vi "getEngineeringStatus.vi"(8 "error in (no error)":errorcluster, 11 "DomeCommunicator in":refnum<class "DomeCommunicator.lvclass">) -> (0 "error out":errorcluster, 1 "timeout":bool, 2 "fullEngineeringStatus":T1 {"shortStatus"."azimuthAngle" min=0.0 max=360.0; "shortStatus"."dropoutDoorOpeningPercentage" min=0.0 max=100.0; "shortStatus"."mainDoorOpeningPercentage" min=0.0 max=100.0}, 3 "DomeCommunicator out":refnum<class "DomeCommunicator.lvclass">, 4 "response":string)   [LabVIEW 2016, in "DomeCommunicator.lvclass"]
uses:
  DomeCommunicator.lvclass
  ComTypedefs/fullEngineeringStatus.ctl
  ComTypedefs/shortStatus.ctl
  ComTypedefs/openingStates.ctl
  IDome/domeTypedefs/openingPercentage.ctl
  ComTypedefs/sensorCode.ctl
  ComTypedefs/azimimuthPositionStatus.ctl
  IDome/domeTypedefs/azimuth.ctl
  IDome/domeTypedefs/direction.ctl
  IDome/domeTypedefs/domeState.ctl
  IDome/domeTypedefs/motionDirection.ctl
  IDome/domeTypedefs/openingMotion.ctl
  ComTypedefs/engineeringStatus.ctl
  ComTypedefs/queries.ctl
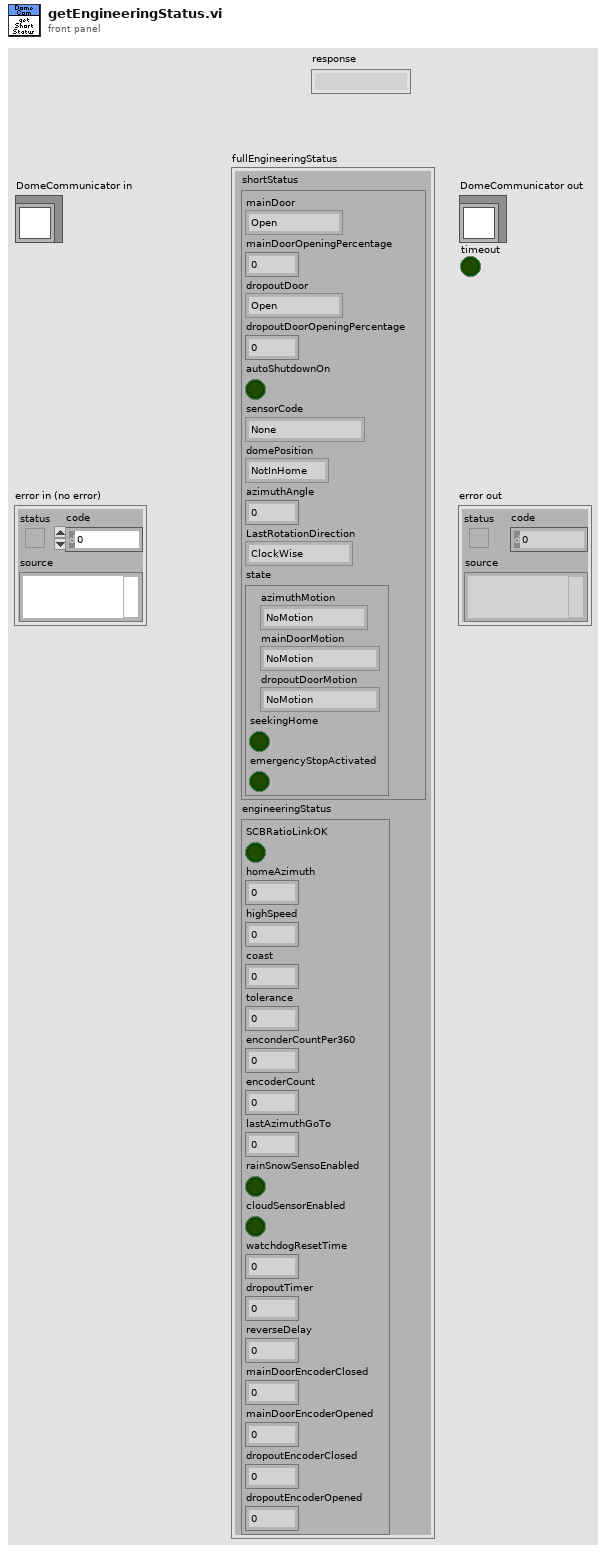
[diagram p1: front panel]
types:
  T1 = typedef "fullEngineeringStatus.ctl" = cluster{"shortStatus":T2, "engineeringStatus":T12}
  T2 = typedef "shortStatus.ctl" = cluster{"mainDoor":T3, "mainDoorOpeningPercentage":T4, "dropoutDoor":T3, "dropoutDoorOpeningPercentage":T4, "autoShutdownOn":bool, "sensorCode":T5, "domePosition":T6, "azimuthAngle":T7, "LastRotationDirection":T8, "state":T9}
  T3 = typedef "openingStates.ctl" = enum16{"Open", "Shut", "Ajar"}
  T4 = typedef "openingPercentage.ctl" = dbl
  T5 = typedef "sensorCode.ctl" = enum16{"None", "RainSnowSensorTriggered", "CloudSensorTriggered", "BothSensorsTriggered"}
  T6 = typedef "azimimuthPositionStatus.ctl" = enum16{"NotInHome", "Home"}
  T7 = typedef "azimuth.ctl" = dbl
  T8 = typedef "direction.ctl" = enum16{"ClockWise", "CounterClockWise"}
  T9 = typedef "domeState.ctl" = cluster{"azimuthMotion":T10, "mainDoorMotion":T11, "dropoutDoorMotion ":T11, "seekingHome":bool, "emergencyStopActivated":bool}
  T10 = typedef "motionDirection.ctl" = enum16{"NoMotion", "MovingClockWise", "MovingCounterClockWise"}
  T11 = typedef "openingMotion.ctl" = enum16{"NoMotion", "Opening", "Closing"}
  T12 = typedef "engineeringStatus.ctl" = cluster{"SCBRatioLinkOK":bool, "homeAzimuth":dbl, "highSpeed":dbl, "coast":dbl, "tolerance":dbl, "enconderCountPer360":u32, "encoderCount":u32, "lastAzimuthGoTo":dbl, "rainSnowSensoEnabled":bool, "cloudSensorEnabled":bool, "watchdogResetTime":dbl, "dropoutTimer":dbl, "reverseDelay":dbl, "mainDoorEncoderClosed":u32, "mainDoorEncoderOpened":u32, "dropoutEncoderClosed":u32, "dropoutEncoderOpened":u32}
  T13 = typedef "queries.ctl" = enum16{"ShortStatus", "FullEngineeringStatus", "RecallLastSavedConfiguration"}
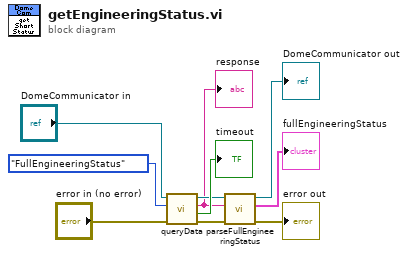
[diagram p0: block diagram]
diagram:
  n1 = call "queryData.vi"("error in (no error)"="error in (no error)", "queries"=queries."FullEngineeringStatus", "DomeCommunicator in"="DomeCommunicator in") -> ("error out"=w4:errorcluster, "timeout"=→"timeout":bool, "response"=w5:string, "DomeCommunicator out"=w6:refnum<class "DomeCommunicator.lvclass">)  [unwired: 5 in]
  "response" <- w5
  n2 = call "parseFullEngineeringStatus.vi"("error in (no error)"=w4, "engineeringStatusString"=w5, "DomeCommunicator in"=w6) -> ("error out"=→"error out":errorcluster, "fullEngineeringStatus"=→"fullEngineeringStatus":T1, "DomeCommunicator out"=→"DomeCommunicator out":refnum<class "DomeCommunicator.lvclass">)  [unwired: 6 in]
